vi "Launcher Main.vi"() -> ()   [LabVIEW 2024]
doc: "ControllerUI API Tester."
uses:
  <vilib>/Utility/error.llb/DialogType.ctl
  Libraries/ControllerUI/ControllerUI.lvlib
  Libraries/Launcher Support/Launcher Support.lvlib
panel:
  in  "Launch Mensajes API Tester":bool
  in  "Launch Product API Tester":bool
  in  "Launch Money API Tester":bool
  out "Command Line Arguments":string[](array[string])
  out "last error":errorcluster
  in  "Show Diagram on Init":bool
  in  "Show Block Diagram":bool
  in  "Stop Module":bool
  in  "Start Module":bool
  in  "Hide Module Panel":bool
  in  "Show Module Panel":bool
  out "Status":string
  out "Module Running?":bool
  # "This VI tests the API for the Module."
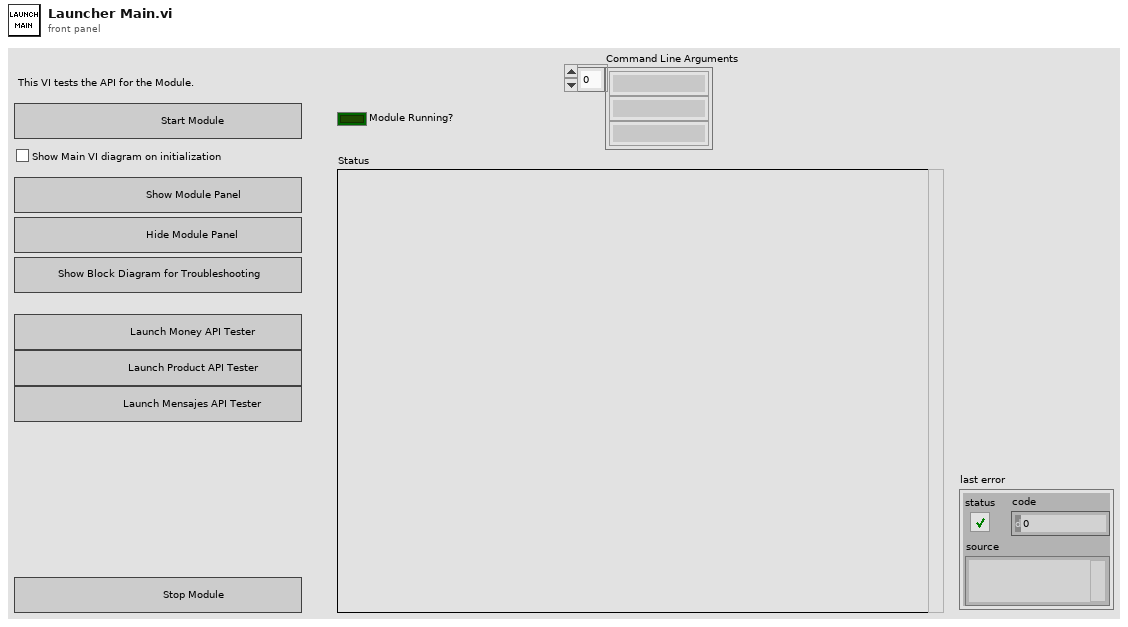
[diagram p1: front panel]
types:
  T1 = enum32{"invalid app kind", "Development System", "Run Time System", "Student Edition", "Embedded LabVIEW", "Evaluation", "Custom"}
  T2 = typedef "ControllerUI.lvlib/Broadcast Events--cluster.ctl" = cluster{"Module Did Init":refnum<user-event>, "Status Updated":refnum<user-event>, "Error Reported":refnum<user-event>, "Module Did Stop":refnum<user-event>, "Update Module Execution Status":refnum<user-event>}
  T3 = typedef "DialogType.ctl" = u16
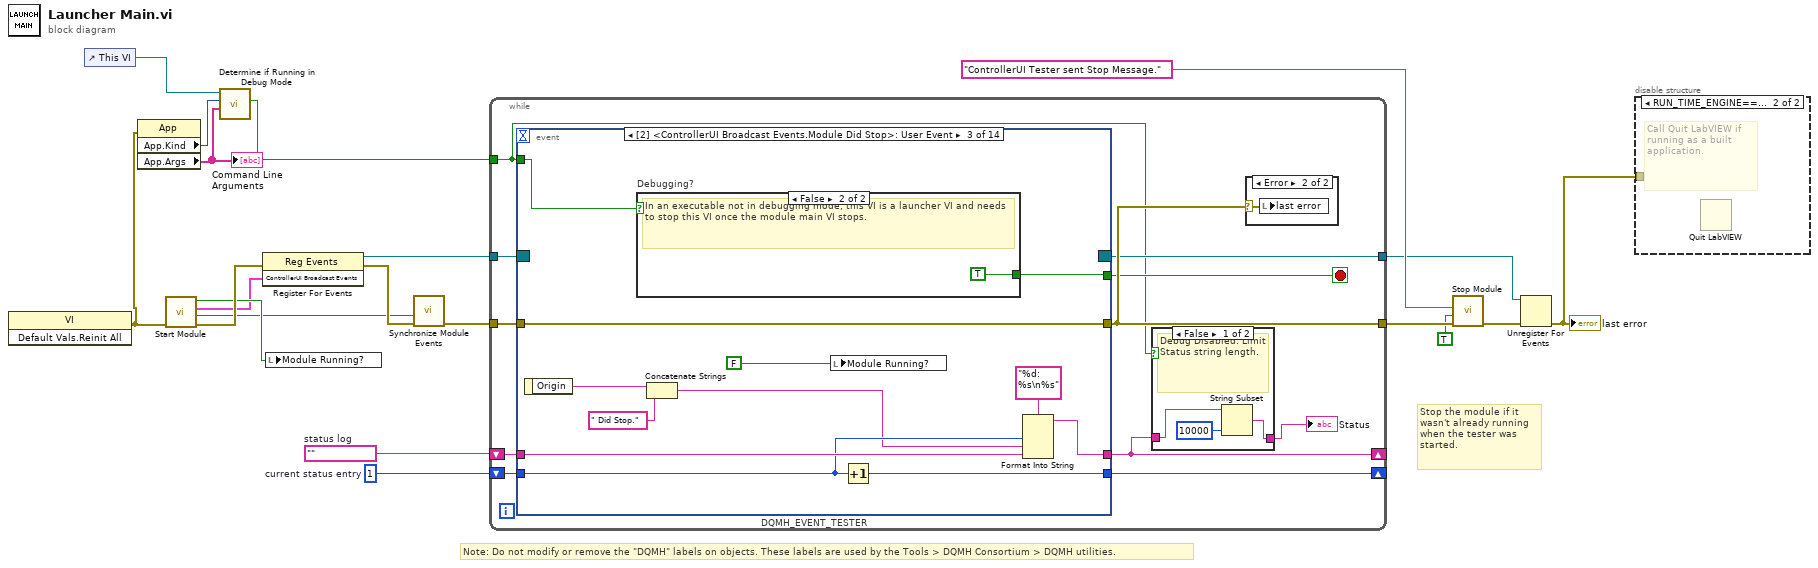
[diagram p0: block diagram]
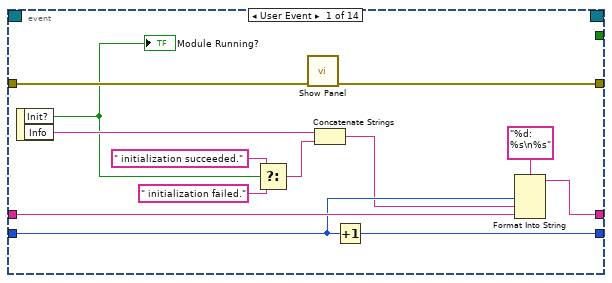
[diagram p5: hidden frame]
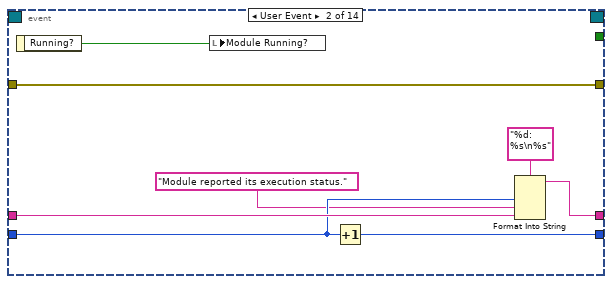
[diagram p6: hidden frame]
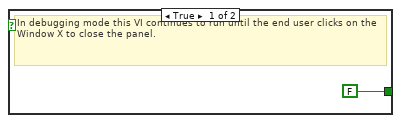
[diagram p7: hidden frame]
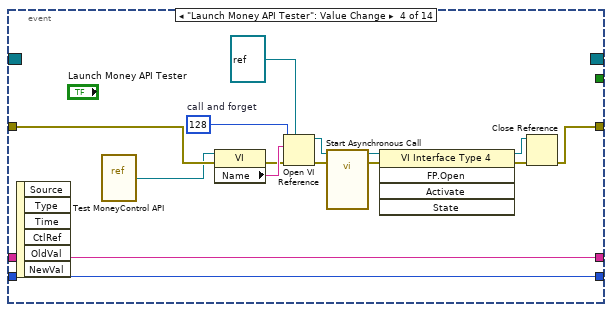
[diagram p8: hidden frame]
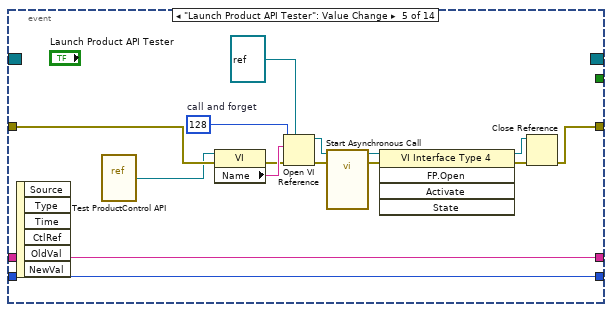
[diagram p9: hidden frame]
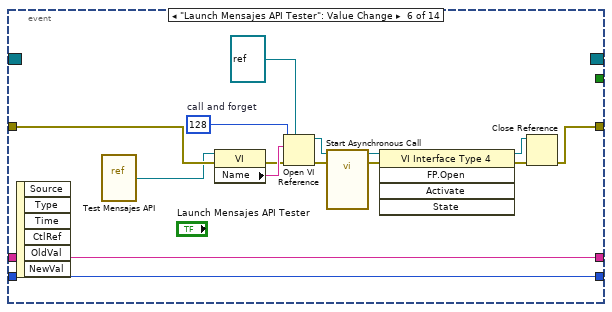
[diagram p10: hidden frame]
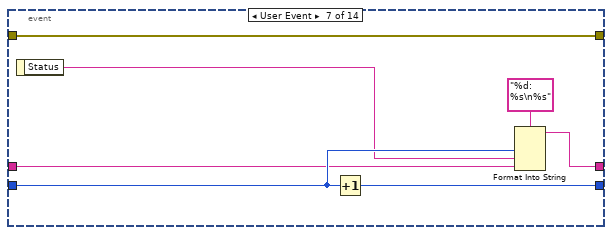
[diagram p11: hidden frame]
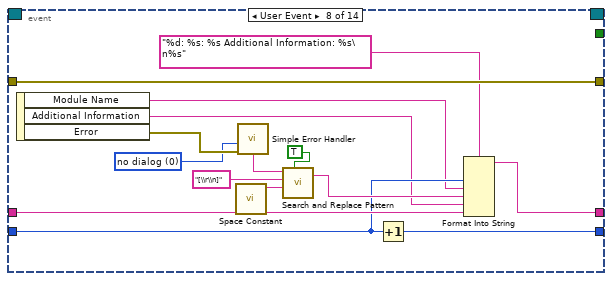
[diagram p12: hidden frame]
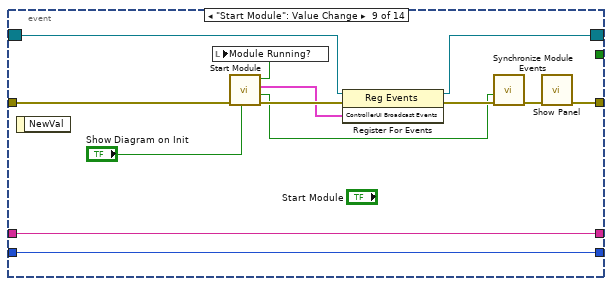
[diagram p13: hidden frame]
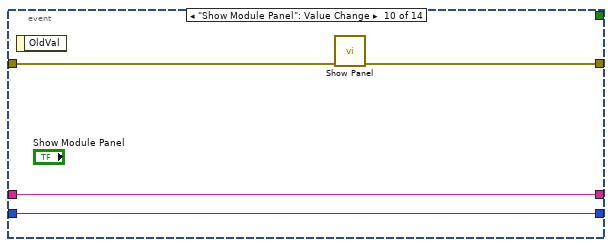
[diagram p14: hidden frame]
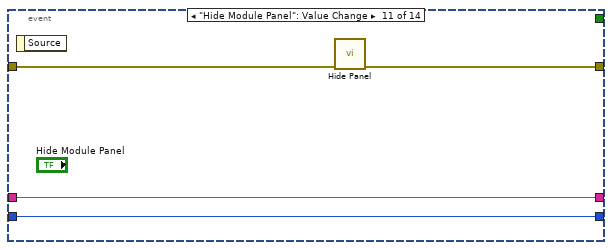
[diagram p15: hidden frame]
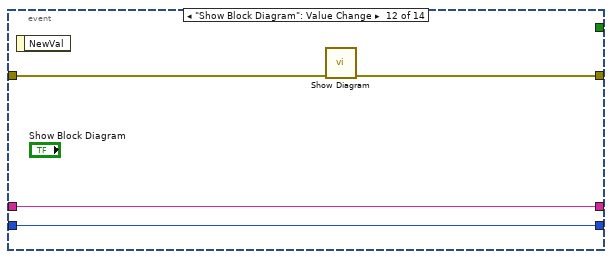
[diagram p16: hidden frame]
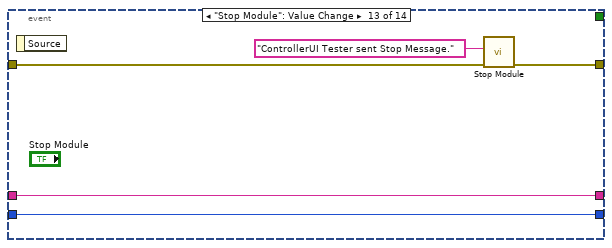
[diagram p17: hidden frame]
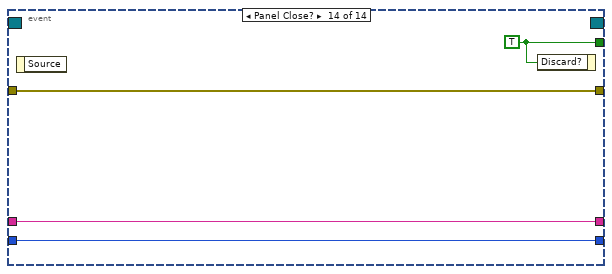
[diagram p18: hidden frame]
diagram:
  w13 = 1  # current status entry
  w14 = ""  # status log
  # "Stop the module if it wasn't already running when the tester was started."
  # "Note: Do not modify or remove the \"DQMH\" labels on objects. These labels are used by the Tools > DQMH Consortium > DQMH utilities."
  n1 = invoke class="VI" method="Default Vals.Reinit All"() -> (error out=w6:errorcluster)  [unwired: 3 in, 2 out]
  n2 = control-ref of="This VI"() -> (w7:refnum<vi>)
  n3 = property on="Property Node" class="App"(error in=w6) -> ("App.Kind"=w5:T1, "App.Args"=w4:string[])  [unwired: 1 in, 2 out]
  "Command Line Arguments" <- w4
  n4 = call "Start Module.vi"("error in"=w6) -> ("error out"=w18:errorcluster, "Wait for Event Sync?"=w8:bool, "ControllerUI Broadcast Events"=w9:T2, "Module Was Already Running?"=w10:bool)  [unwired: 6 in, 1 out]
  n5 = call "Determine if Running in Debug Mode.vi"("App.Args"=w4, "App.Kind"=w5, "Launcher VI ref"=w7) -> ("Debug mode?"=w3:bool)  [unwired: 8 in]
  n6 = register-events(error in=w18, w9) -> (reference out=w12:refnum<event-registration>, error out=w17:errorcluster)  [unwired: 1 in]
  n7 = local write "Module Running?"(w10) -> ()
  n8 = call "Synchronize Module Events.vi"("error in"=w17, "Wait for Event Sync?"=w8) -> ("error out"=w16:errorcluster)  [unwired: 9 in]
  n9 = while {
    tunnel: w12 -> [w29]
    tunnel: [w30] -> w19
    shift-right: [w23] -> _
    shift-left: w14 -> [w27]
    shift-right: [w26] -> _
    shift-left: w13 -> [w28]
    tunnel: w16 -> [w31]
    tunnel: [w25] -> w11
    tunnel: w3 -> [w21]
    stop <- w24 stop-if-true
    n10 = event "DQMH_EVENT_TESTER" shown="[2] <ControllerUI Broadcast Events.Module Did Stop>: User Event" {
      selector: w29 -> [_ _ _ _ _ _ _ _ w142 _ _ _ _ _]
      dyn-events: [_ _ _ _ _ _ _ _ w141 _ _ _ _ _] -> w25
      timeout: _ -> [_ _ _ _ _ _ _ _ _ _ _ _ _ _]
      tunnel: [_ _ w59 _ _ _ _ _ _ _ _ _ _ w171] -> w24
      tunnel: [w48 w57 w69 w74 w89 w104 w123 w138 w147 w155 w159 w162 w168 w172] -> w30
      tunnel: w28 -> [w45 w54 w66 w85 w100 w115 w119 w128 w145 w152 w156 w160 w165 w169]
      tunnel: w27 -> [w46 w55 w67 w86 w101 w116 w118 w129 w146 w153 w157 w161 w166 w170]
      tunnel: [w43 w52 w64 w86 w101 w116 w120 w127 w146 w153 w157 w161 w166 w170] -> w23
      tunnel: [w44 w53 w65 w85 w100 w115 w122 w126 w145 w152 w156 w160 w165 w169] -> w26
      tunnel: w31 -> [w49 w57 w69 w73 w88 w103 w123 w138 w149 w154 w158 w163 w167 w172]
      tunnel: w21 -> [_ _ w58 _ _ _ _ _ _ _ _ _ _ _]
      event User Event {
        n11 = event-data() -> ("Init?"=w40:bool, "Info"=w42:string)  [unwired: 1 in]
        "Module Running?" <- w40
        n12 = Select(t=" initialization succeeded.", s=w40, f=" initialization failed.") -> (s? t:f=w37:string)
        n13 = call "Show Panel.vi"("error in"=w49) -> ("error out"=w48:errorcluster)  [unwired: 10 in]
        n14 = Concatenate Strings(w42, w37) -> (w41:string)
        n15 = Increment(x=w45) -> (x+1=w44:i32)
        n16 = Format Into String(format string="%d: %s\n%s", w45, w41, w46) -> (resulting string=w43:string)  [unwired: 2 in, 1 out]
      }
      event User Event {
        n17 = event-data() -> ("Running?"=w50:bool)  [unwired: 1 in]
        n18 = local write "Module Running?"(w50) -> ()
        n19 = Increment(x=w54) -> (x+1=w53:i32)
        n20 = Format Into String(format string="%d: %s\n%s", w54, "Module reported its execution status.", w55) -> (resulting string=w52:string)  [unwired: 2 in, 1 out]
      }
      event User Event {
        n21 = event-data() -> ("Origin"=w63:string)  [unwired: 1 in]
        n22 = case "Debugging?" shown="False" w58 {
          tunnel: [FALSE ("Discard?") TRUE ("Discard?")] -> w59
          frame True {
            # "In debugging mode this VI continues to run until the end user clicks on the Window X to close the panel."
          }
          frame False {
            # "In an executable not in debugging mode, this VI is a launcher VI and needs to stop this VI once the module main VI stops."
          }
        }
        n23 = Concatenate Strings(w63, " Did Stop.") -> (w62:string)
        n24 = local write "Module Running?"(FALSE ("Module Did Init?")) -> ()
        n25 = Increment(x=w66) -> (x+1=w65:i32)
        n26 = Format Into String(format string="%d: %s\n%s", w66, w62, w67) -> (resulting string=w64:string)  [unwired: 2 in, 1 out]
      }
      event "Launch Money API Tester": Value Change {
        w75 = 128  # call and forget
        n27 = event-data() -> ()  [unwired: 1 in, 6 out]
        n28 = vi-ref "Test MoneyControl API.vi"() -> (w72:refnum<vi>)
        n29 = property class="VI"(reference=w72, error in=w73) -> (error out=w77:errorcluster, "Name"=w79:string)  [unwired: 1 out]
        n30 = Open VI Reference(type specifier VI Refnum (for type only)=refnum<vi> refnum, vi path=w79, options=w75, error in (no error)=w77) -> (vi reference=w81:refnum<vi>, error out=w78:errorcluster)  [unwired: 2 in]
        n31 = call-by-ref "Start Asynchronous Call"(reference=w81, error in=w78) -> (reference out=w83:refnum<vi>, error out=w80:errorcluster)  [unwired: 12 in]
        n32 = invoke class="VI Interface Type 4" method="FP.Open"(reference=w83, error in=w80) -> (reference out=w84:refnum<vi>, error out=w82:errorcluster)  [unwired: 3 in, 3 out]
        n33 = Close Reference(reference=w84, error in (no error)=w82) -> (error out=w74:errorcluster)
      }
      event "Launch Product API Tester": Value Change {
        w90 = 128  # call and forget
        n34 = event-data() -> ()  [unwired: 1 in, 6 out]
        n35 = vi-ref "Test ProductControl API.vi"() -> (w87:refnum<vi>)
        n36 = property class="VI"(reference=w87, error in=w88) -> (error out=w92:errorcluster, "Name"=w94:string)  [unwired: 1 out]
        n37 = Open VI Reference(type specifier VI Refnum (for type only)=refnum<vi> refnum, vi path=w94, options=w90, error in (no error)=w92) -> (vi reference=w96:refnum<vi>, error out=w93:errorcluster)  [unwired: 2 in]
        n38 = call-by-ref "Start Asynchronous Call"(reference=w96, error in=w93) -> (reference out=w98:refnum<vi>, error out=w95:errorcluster)  [unwired: 12 in]
        n39 = invoke class="VI Interface Type 4" method="FP.Open"(reference=w98, error in=w95) -> (reference out=w99:refnum<vi>, error out=w97:errorcluster)  [unwired: 3 in, 3 out]
        n40 = Close Reference(reference=w99, error in (no error)=w97) -> (error out=w89:errorcluster)
      }
      event "Launch Mensajes API Tester": Value Change {
        w105 = 128  # call and forget
        n41 = event-data() -> ()  [unwired: 1 in, 6 out]
        n42 = vi-ref "Test Mensajes API.vi"() -> (w102:refnum<vi>)
        n43 = property class="VI"(reference=w102, error in=w103) -> (error out=w107:errorcluster, "Name"=w109:string)  [unwired: 1 out]
        n44 = Open VI Reference(type specifier VI Refnum (for type only)=refnum<vi> refnum, vi path=w109, options=w105, error in (no error)=w107) -> (vi reference=w111:refnum<vi>, error out=w108:errorcluster)  [unwired: 2 in]
        n45 = call-by-ref "Start Asynchronous Call"(reference=w111, error in=w108) -> (reference out=w113:refnum<vi>, error out=w110:errorcluster)  [unwired: 12 in]
        n46 = invoke class="VI Interface Type 4" method="FP.Open"(reference=w113, error in=w110) -> (reference out=w114:refnum<vi>, error out=w112:errorcluster)  [unwired: 3 in, 3 out]
        n47 = Close Reference(reference=w114, error in (no error)=w112) -> (error out=w104:errorcluster)
      }
      event User Event {
        n48 = event-data() -> ("Status"=w117:string)  [unwired: 1 in]
        n49 = Increment(x=w119) -> (x+1=w122:i32)
        n50 = Format Into String(format string="%d: %s\n%s", w119, w117, w118) -> (resulting string=w120:string)  [unwired: 2 in, 1 out]
      }
      event User Event {
        w130 = T3 0 items=["no dialog", "OK message", "continue or stop message", "OK message + warnings", "continue/stop + warnings"] ("type of dialog (OK msg:1)")
        n51 = event-data() -> ("Module Name"=w125:string, "Additional Information"=w124:string, "Error"=w137:errorcluster)  [unwired: 1 in]
        n52 = call <vilib>:"Space Constant.vi"() -> ("String"=w134:string)
        n53 = call <vilib>:"Simple Error Handler.vi"("type of dialog (OK msg:1)"=w130, "error in (no error)"=w137) -> ("message"=w131:string)  [unwired: 3 in, 4 out]
        n54 = call <vilib>:"Search and Replace Pattern.vi"("string"=w131, "regular expression (\"\")"="[\\r\\n]" ("regular expression (\"\")"), "replace string (\"\")"=w134, "replace all? (F)"=TRUE ("replace all CR/LF with spaces")) -> ("result string"=w132:string)  [unwired: 1 in, 1 out]
        n55 = Increment(x=w128) -> (x+1=w126:i32)
        n56 = Format Into String(format string="%d: %s: %s Additional Information: %s\n%s", w128, w125, w132, w124, w129) -> (resulting string=w127:string)  [unwired: 2 in, 1 out]
      }
      event "Start Module": Value Change {
        n57 = event-data() -> ()  [unwired: 1 in, 1 out]
        n58 = call "Start Module.vi"("Show Main VI Diagram on Init (F)"="Show Diagram on Init", "error in"=w149) -> ("error out"=w150:errorcluster, "Wait for Event Sync?"=w144:bool, "ControllerUI Broadcast Events"=w143:T2, "Module Was Already Running?"=w140:bool)  [unwired: 5 in, 1 out]
        n59 = local write "Module Running?"(w140) -> ()
        n60 = register-events(reference=w142, error in=w150, w143) -> (reference out=w141:refnum<event-registration>, error out=w151:errorcluster)
        n61 = call "Synchronize Module Events.vi"("error in"=w151, "Wait for Event Sync?"=w144) -> ("error out"=w148:errorcluster)  [unwired: 9 in]
        n62 = call "Show Panel.vi"("error in"=w148) -> ("error out"=w147:errorcluster)  [unwired: 10 in]
      }
      event "Show Module Panel": Value Change {
        n63 = event-data() -> ()  [unwired: 1 in, 1 out]
        n64 = call "Show Panel.vi"("error in"=w154) -> ("error out"=w155:errorcluster)  [unwired: 10 in]
      }
      event "Hide Module Panel": Value Change {
        n65 = event-data() -> ()  [unwired: 1 in, 1 out]
        n66 = call "Hide Panel.vi"("error in"=w158) -> ("error out"=w159:errorcluster)  [unwired: 10 in]
      }
      event "Show Block Diagram": Value Change {
        n67 = event-data() -> ()  [unwired: 1 in, 1 out]
        n68 = call "Show Diagram.vi"("error in"=w163) -> ("error out"=w162:errorcluster)  [unwired: 10 in]
      }
      event "Stop Module": Value Change {
        n69 = event-data() -> ()  [unwired: 1 in, 1 out]
        n70 = call "Stop Module.vi"("error in"=w167, "Origin"="ControllerUI Tester sent Stop Message.") -> ("error out"=w168:errorcluster)  [unwired: 9 in]
      }
      event Panel Close? {
        w171 = TRUE ("Discard?")
        n71 = event-data() -> ()  [unwired: 1 in, 1 out]
        n72 = event-data("Discard?"=w171) -> ()  [unwired: 1 in, 1 out]
      }
    }
    n73 = case shown="False" w21 {
      tunnel: w23 -> [w34 w35]
      tunnel: [w33 w35] -> w22
      frame False {
        # "Debug Disabled. Limit Status string length."
        n74 = String Subset(string=w34, length (rest)=10000 ("length (rest)")) -> (substring=w33:string)  [unwired: 1 in]
      }
      frame True {
        # "Debug Enabled. Do not limit Status string length."
      }
    }
    "Status" <- w22
    n75 = case shown="Error" w30 {
      selector: w30 -> [_ w36]
      frame No Error {
      }
      frame Error {
        n76 = local write "last error"(w36) -> ()
      }
    }
  }
  n77 = call "Stop Module.vi"("error in"=w19, "Wait for Module to Stop? (F)"=TRUE ("Wait for Module to stop?"), "Origin"="ControllerUI Tester sent Stop Message.") -> ("error out"=w20:errorcluster)  [unwired: 8 in]
  n78 = Unregister For Events(event registration refnum=w11, error in=w20) -> (error out=w1:errorcluster)
  "last error" <- w1
  n79 = disable-structure "Conditional Disable Structure" shown="RUN_TIME_ENGINE==True" {
    disable-tunnel: w1 -> [_ _]
    frame condition #0 (active) {
    }
    frame condition #1 {
      # "Call Quit LabVIEW if running as a built application."
      n80 = Quit LabVIEW() -> ()  [unwired: 1 in]
    }
  }
